vi "DMR_Init.vi"() -> (1 "handle device manager OUT":i32, 2 "error code OUT":i32)   [LabVIEW 2016]
doc: "Initialises the device manager.\n\nThis VI initialises internal data structures and locates devices and device driver in the system.\n\nBefore any device can be accessed the user MUST successfully call this VI.\nDMR_Init can be called multiple times, but for each call to this function a call to DMR_Close must be executed before ending the application as otherwise resource leaks will occur.\n\nIf this function is called multiple times in the same process without calling DMR_Close in between no additional work is performed by the function, but an internal usage counter \nis incremented.\n\nSee also:\nDMR_Close()\n \nThe 'error code OUT' terminal will deliver 0 if successful or a negative error code otherwise. A list of valid error codes and their meaning can be found in the manual about this interface.\n\nThe other output receives a handle to the device manager, but this parameter is currently unsupported."
uses:
  mvDeviceManager.dll
panel:
  # "OUTPUT"
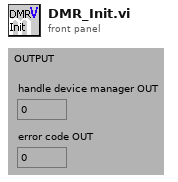
[diagram p1: front panel]
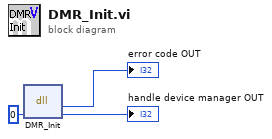
[diagram p0: block diagram]
diagram:
  n1 = dll-call lib="mvDeviceManager.dll" fn="DMR_Init"(0 ("Eingangswert")) -> (→"error code OUT":i32, →"handle device manager OUT":i32)  [unwired: 3 in, 2 out]
